vi "SwerveDriveCalibrate.vi"() -> ()   [LabVIEW 2014]
uses:
  <vilib>/Platform/TimedLoop/XDataNode/timing_clust.ctl
  <vilib>/Platform/TimedLoop/XDataNode/nitl_modes.ctl
  <vilib>/Platform/TimedLoop/XDataNode/wakeup.ctl
  <vilib>/Rock Robotics/WPI/CAN/TalonSRX/WPI_CANTalonSRX_APIControlMode.ctl
  <vilib>/Rock Robotics/WPI/CAN/TalonSRX/WPI_CANTalonSRX_APIFeedbackSelect.ctl
  <vilib>/Rock Robotics/WPI/SafetyOutput/WPI_SafetyOutputConfigMenu.ctl
  <vilib>/Rock Robotics/WPI/MotorControl/WPI_MotorControlOpenCANTalonSRX.vi
  <vilib>/Platform/TimedLoop/XDataNode/XDataNode.xnode
  <vilib>/Rock Robotics/WPI/MotorControl/WPI_MotorControlType.ctl
  <vilib>/Rock Robotics/SystemInterfaces/Typedef/FPGA_TypedefDigitalModule.ctl
  <vilib>/Rock Robotics/SystemInterfaces/DIO/FPGA_DIOPWMChannel.ctl
  <vilib>/Rock Robotics/WPI/PWM/WPI_PWMDeadband.ctl
  <vilib>/Rock Robotics/WPI/CAN/Jaguar/SubVIs/WPI_CANJaguar_ControlMode.ctl
  <vilib>/Rock Robotics/WPI/PWM/WPI_PWMTransform_ConPane.ctl
  <vilib>/Rock Robotics/WPI/MotorControl/WPI_MotorControlDeviceRef.ctl
  <vilib>/Platform/TimedLoop/XDataNode/XDNodeRunTimeDep.lvlib
panel:
  out "Analog In":dbl
  out "Encoder Position (-SRX)":dbl
  out "Sensor Position":dbl
  out "Quad velocities":dbl[](array[numeric])
  in  "Speed %VBus":dbl(slide) scale=-0.5..0.5
  out "Wheel Position":dbl(knob) scale=3.1416..-3.1416
  in  "Motor Controller":T1(ring)
  out "Waveform Chart":cluster{dbl, "motor output angle":dbl}(graph)
  in  "Enable":bool
  in  "Target Angle":dbl(knob) scale=3.1416..-3.1416
  in  "Offset":dbl
  in  "TPR":dbl=162.974661726
  in  "Set":bool
  in  "stop":bool
  out "error out":errorcluster
  in  "Steering PID":cluster{"P":dbl, "I":dbl, "D":dbl}
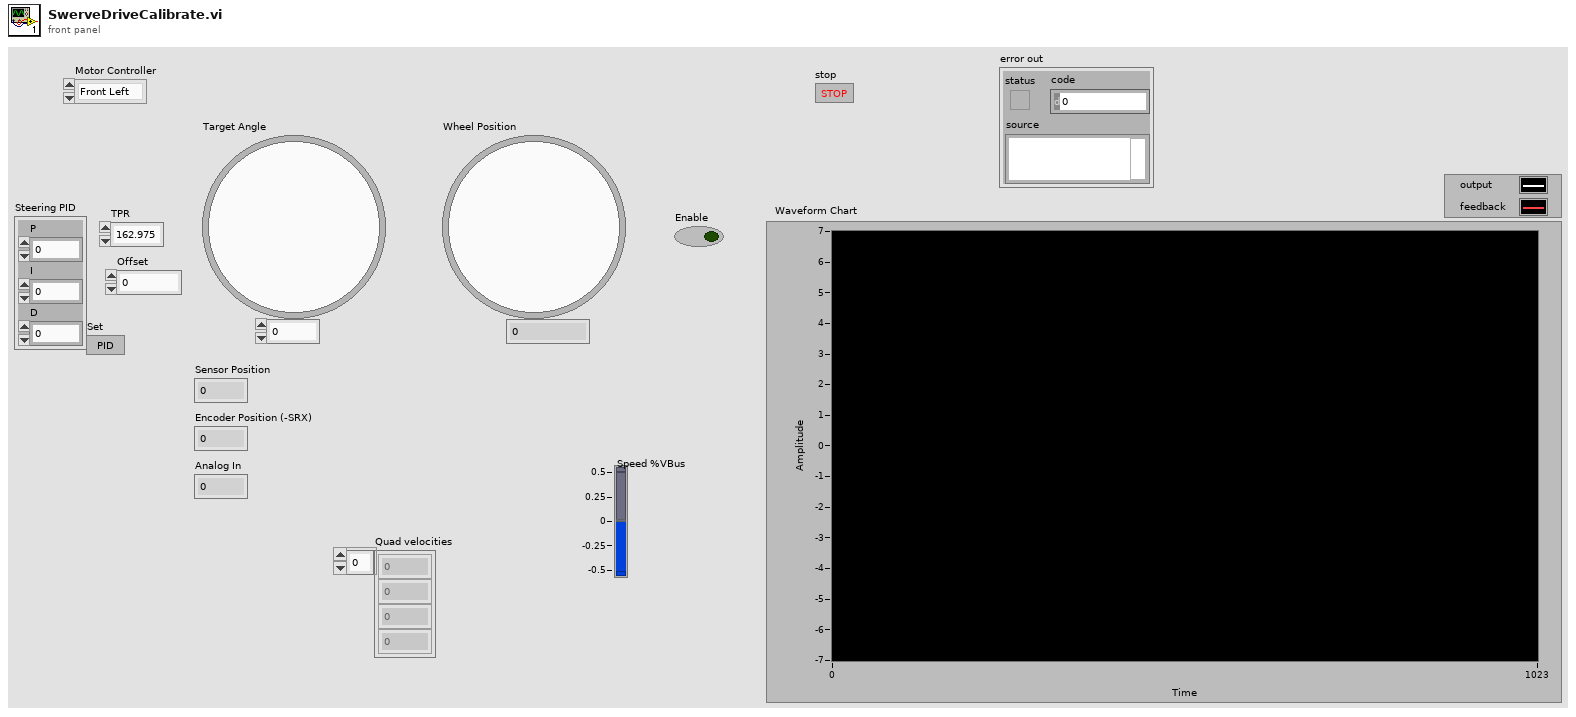
[diagram p1: front panel]
types:
  T1 = enum16{"Front Left", "Front Right", "Rear Left", "Rear Right"}
  T2 = typedef "WPI_MotorControlDeviceRef.ctl" = cluster{"DeviceStatus":errorcluster, "Type":T3, "PWM":cluster{"Controller":T4, "PWM Channel":T5, "DeadBand":T6}, "CAN":cluster{"Device Number":u8, "Control Mode":T7, "Semaphore":T8, "Max Vout":dbl, "TalonSRX Control Mode":T9}, "Invert":bool, "TransformRef":T10, "InvTransformRef":T10}
  T3 = typedef "WPI_MotorControlType.ctl" = enum16{"PWM", "CAN", "CANTalonSRX"}
  T4 = typedef "FPGA_TypedefDigitalModule.ctl" = enum16{"Controller 1"}
  T5 = typedef "FPGA_DIOPWMChannel.ctl" = enum8{"PWM 0", "PWM 1", "PWM 2", "PWM 3", "PWM 4", "PWM 5", "PWM 6", "PWM 7", "PWM 8", "PWM 9", "PWM MXP 0", "PWM MXP 1", "PWM MXP 2", "PWM MXP 3", "PWM MXP 4", "PWM MXP 5", "PWM MXP 6", "PWM MXP 7", "PWM MXP 8", "PWM MXP 9", "Invalid"}
  T6 = typedef "WPI_PWMDeadband.ctl" = cluster{"Name":string, "maxPositivePwm":i32, "minPositivePwm":i32, "centerPwm":i32, "maxNegativePwm":i32, "minNegativePwm":i32, "angularRange":u16}
  T7 = typedef "WPI_CANJaguar_ControlMode.ctl" = enum8{"Percent VBus", "Current", "Speed", "Position", "Voltage"}
  T8 = typedef "Semaphore RefNum" = refnum<k1>
  T9 = typedef "WPI_CANTalonSRX_APIControlMode.ctl" = enum8{"Percent VBus", "Speed", "Position", "Slave", "Unchanged / Invalid"}
  T10 = typedef "WPI_PWMTransform_ConPane.ctl" = refnum<vi>
  T11 = typedef "WPI_CANTalonSRX_APIFeedbackSelect.ctl" = enum16{"Digital Quadrature Encoder", "Analog Potentiometer", "Analog Encoder"}
  T12 = typedef "WPI_SafetyOutputConfigMenu.ctl" = enum16{"Enable", "Disable"}
  T13 = typedef "WPI_CANTalonSRX_GlobalStatus.ctl" = cluster{"Applied Throttle":dbl, "Module Enabled":bool, "CAN Error":errorcluster, "Closed Loop Error":dbl, "Forward Limit Switch Closed":bool, "Reverse Limit Switch Closed":bool, "Sensor Position":dbl, "Sensor Velocity":dbl, "Current":dbl, "Sticky Fault - Over Temp":bool, "Sticky Fault - Under Voltage":bool, "Sticky Fault - Forward Limit":bool, "Sticky Fault - Reverse Limit":bool, "Sticky Fault - Forward Soft Limit":bool, "Sticky Fault - Reverse Soft Limit":bool, "Brake is Enabled":bool, "Encoder Position":dbl, "Encoder Velocity":dbl, "Encoder Index Count":dbl, "Encoder A Pin State":bool, "Encoder B Pin State":bool, "Encoder Index Pin State":bool, "Analog In":dbl, "Analog In Velocity":dbl, "Temperature (C)":dbl, "Battery Voltage":dbl}
  T14 = typedef "XDNodeRunTimeDep.lvlib/timing_clust.ctl" = cluster{"Expected End [f-1]":u64, "Actual End [f-1]":u64, "Finished Late? [f-1]":bool, "Expected End [i-1]":u64, "Actual End [i-1]":u64, "Finished Late? [i-1]":bool, "Expected Start [i]":u64, "Actual Start [i]":u64, "Expected Start [f]":u64, "Actual Start [f]":u64, "Source Name":string, "Structure Name":string, "Period":i64, "Deadline":i64, "Offset":i64, "Start":i64, "Priority":i32, "Timeout":i32, "Mode":T15, "Wakeup Reason":T16, "Error":errorcluster, "Source Type":string, "Secondary Source Type":string, "Global End Time":u64, "Global Start Time":u64, "Frame Duration":u64, "Iteration Duration":u64, "Assigned CPU":i32, "I/O Scan Engine Mode":u32}
  T15 = typedef "XDNodeRunTimeDep.lvlib/nitl_modes.ctl" = enum32{"No Change", "Process missed periods, maintain original phase", "Discard missed periods, maintain original phase", "Process missed periods, ignore original phase", "Discard missed periods, ignore original phase"}
  T16 = typedef "XDNodeRunTimeDep.lvlib/wakeup.ctl" = enum32{"Normal", "Aborted", "Asynchronous wakeup", "Timing source error", "Timed loop error", "Timeout"}
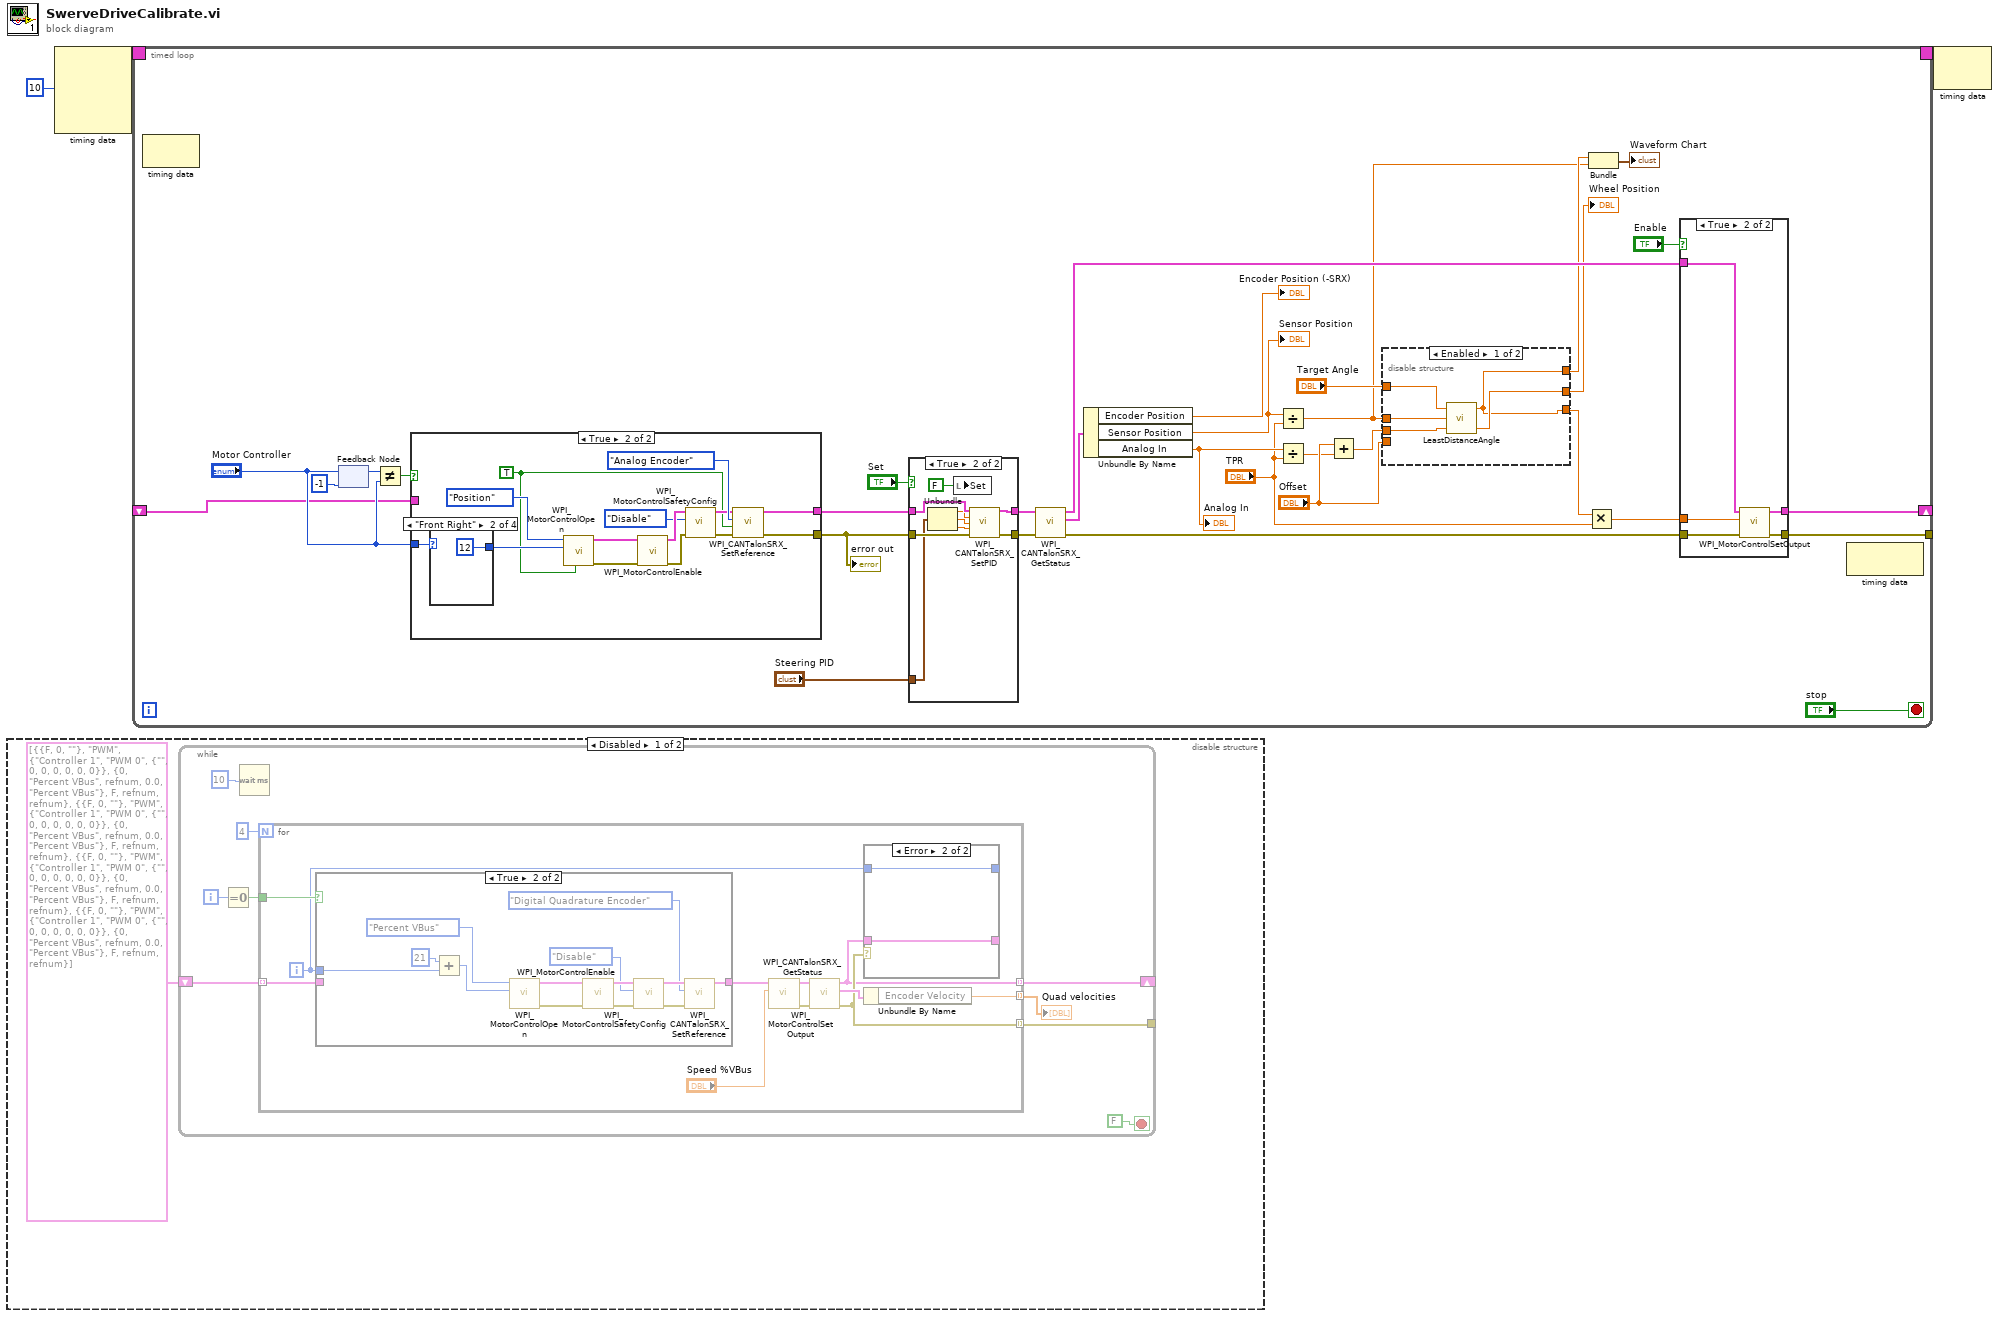
[diagram p0: block diagram]
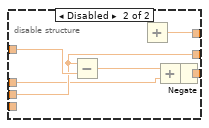
[diagram p5: hidden frame]
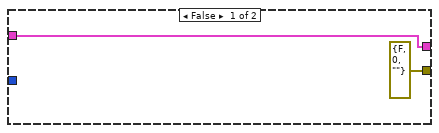
[diagram p6: hidden frame]
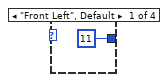
[diagram p7: hidden frame]
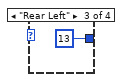
[diagram p8: hidden frame]
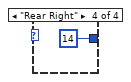
[diagram p9: hidden frame]
diagram:
  n1 = disable-structure shown="Disabled" {
    frame Disabled {
      n2 = while {
        shift-right: [w9] -> _
        shift-left: T2[] [{"DeviceStatus"={"status"=FALSE, "code"=0, "source"=""}, "Type"=enum."PWM", "PWM"={"Controller"=enum."Controller 1", "PWM Channel"=enum."PWM 0", "DeadBand"={"Name"="", "maxPositivePwm"=0, "minPositivePwm"=0, "centerPwm"=0, "maxNegativePwm"=0, "minNegativePwm"=0, "angularRange"=0}}, "CAN"={"Device Number"=0, "Control Mode"=enum."Percent VBus", "Semaphore"=refnum, "Max Vout"=0.0, "TalonSRX Control Mode"=enum."Percent VBus"}, "Invert"=FALSE, "TransformRef"=refnum, "InvTransformRef"=refnum}, {"DeviceStatus"={"status"=FALSE, "code"=0, "source"=""}, "Type"=enum."PWM", "PWM"={"Controller"=enum."Controller 1", "PWM Channel"=enum."PWM 0", "DeadBand"={"Name"="", "maxPositivePwm"=0, "minPositivePwm"=0, "centerPwm"=0, "maxNegativePwm"=0, "minNegativePwm"=0, "angularRange"=0}}, "CAN"={"Device Number"=0, "Control Mode"=enum."Percent VBus", "Semaphore"=refnum, "Max Vout"=0.0, "TalonSRX Control Mode"=enum."Percent VBus"}, "Invert"=FALSE, "TransformRef"=refnum, "InvTransformRef"=refnum}, {"DeviceStatus"={"status"=FALSE, "code"=0, "source"=""}, "Type"=enum."PWM", "PWM"={"Controller"=enum."Controller 1", "PWM Channel"=enum."PWM 0", "DeadBand"={"Name"="", "maxPositivePwm"=0, "minPositivePwm"=0, "centerPwm"=0, "maxNegativePwm"=0, "minNegativePwm"=0, "angularRange"=0}}, "CAN"={"Device Number"=0, "Control Mode"=enum."Percent VBus", "Semaphore"=refnum, "Max Vout"=0.0, "TalonSRX Control Mode"=enum."Percent VBus"}, "Invert"=FALSE, "TransformRef"=refnum, "InvTransformRef"=refnum}, {"DeviceStatus"={"status"=FALSE, "code"=0, "source"=""}, "Type"=enum."PWM", "PWM"={"Controller"=enum."Controller 1", "PWM Channel"=enum."PWM 0", "DeadBand"={"Name"="", "maxPositivePwm"=0, "minPositivePwm"=0, "centerPwm"=0, "maxNegativePwm"=0, "minNegativePwm"=0, "angularRange"=0}}, "CAN"={"Device Number"=0, "Control Mode"=enum."Percent VBus", "Semaphore"=refnum, "Max Vout"=0.0, "TalonSRX Control Mode"=enum."Percent VBus"}, "Invert"=FALSE, "TransformRef"=refnum, "InvTransformRef"=refnum}] -> [w8]
        tunnel: [w6] -> _
        i -> [w12]
        stop <- FALSE stop-if-true
        n3 = Equal To 0?(x=w12) -> (x = 0?=w10:bool)
        n4 = Wait (ms)(milliseconds to wait=u32 10) -> ()  [unwired: 1 out]
        n5 = for {
          N: 4 -> [_]
          tunnel: w10 -> [w24]
          tunnel: [w14] -> w9 mode=indexing
          tunnel: w8 -> [w23] mode=indexing
          tunnel: [w16] -> w6 mode=indexing
          tunnel: [w17] -> w5 mode=indexing
          i -> [w15]
          n6 = case shown="True" w24 {
            tunnel: [w29 w31] -> w22
            tunnel: w23 -> [w29 _]
            tunnel: w15 -> [_ w35]
            frame False {
            }
            frame True {
              n7 = Add(x=21, y=w35) -> (x+y=w34:i32)
              n8 = call-poly <vilib>:"WPI_MotorControlOpen.vi"("Device Number"=w34, "Control Mode"=WPI_CANTalonSRX_APIControlMode."Percent VBus") -> ("error out"=w41:errorcluster, "MotorControlDeviceRef"=w40:T2)  [unwired: 8 in]
              n9 = call <vilib>:"WPI_MotorControlEnable.vi"("error in (no error)"=w41, "CAN Jaguar Ref"=w40) -> ("error out"=w38:errorcluster, "CAN Jaguar Ref Out"=w39:T2)  [unwired: 8 in]
              n10 = call <vilib>:"WPI_MotorControlSafetyConfig.vi"("error in (no error)"=w38, "mode"=WPI_SafetyOutputConfigMenu."Disable", "MotorControlDevRef"=w39) -> ("error out"=w32:errorcluster, "MotorControlDevRef"=w33:T2)  [unwired: 7 in]
              n11 = call <vilib>:"WPI_CANTalonSRX_SetReference.vi"("error in (no error)"=w32, "Feedback Reference"=WPI_CANTalonSRX_APIFeedbackSelect."Digital Quadrature Encoder", "CAN Talon SRX Ref"=w33) -> ("CAN Talon SRX Ref Out"=w31:T2)  [unwired: 7 in, 1 out]
            }
          }
          n12 = call <vilib>:"WPI_MotorControlSetOutput.vi"("Output"="Speed %VBus", "MotorControlDevRef"=w22) -> ("error out"=w20:errorcluster, "MotorControlDevRef"=w19:T2)  [unwired: 7 in, 1 out]
          n13 = call <vilib>:"WPI_CANTalonSRX_GetStatus.vi"("error in (no error)"=w20, "CAN Talon SRX Ref"=w19) -> ("error out"=w16:errorcluster, "Talon SRX Status"=w18:T13, "CAN Talon SRX Ref Out"=w14:T2)  [unwired: 7 in]
          n14 = case shown="Error" w16 {
            tunnel: [w26 w27] -> _
            tunnel: w15 -> [w26 w27]
            tunnel: [w25 w28] -> _
            tunnel: w14 -> [w25 w28]
            frame No Error {
            }
            frame Error {
            }
          }
          n15 = Unbundle By Name(w18) -> ("Encoder Velocity"=w17:dbl)
        }
        "Quad velocities" <- w5
      }
    }
    frame Enabled {
    }
  }
  n16 = node-c288(i64 10 ("Period")) -> (w3:T14)  [unwired: 3 in]
  n17 = timed-loop {
    timing: w3 -> [_]
    timing-out: [_] -> w2
    shift-right: [w62] -> _
    shift-left: _ -> [w54]
    tunnel: [w49] -> _
    stop <- "stop" stop-if-true
    n18 = node-c288() -> ()  [unwired: 1 in, 1 out]
    n19 = feedback-in #1("Motor Controller") -> ()
    n20 = feedback #1(-1) -> (w59:i32)
    n21 = Not Equal?(x=w59, y="Motor Controller") -> (x != y?=w56:bool)
    n22 = case shown="True" w56 {
      tunnel: "Motor Controller" -> [_ w97]
      tunnel: [w88 w96] -> w61
      tunnel: [errorcluster {"status"=FALSE, "code"=0, "source"=""} ("error out") w95] -> w60
      tunnel: w54 -> [w88 _]
      frame False {
      }
      frame True {
        w89 = TRUE ("Invert")
        n23 = case shown="\"Front Right\"" w97 {
          tunnel: [11 12 13 14] -> w99
          frame "Front Left", Default {
          }
          frame "Front Right" {
          }
          frame "Rear Left" {
          }
          frame "Rear Right" {
          }
        }
        n24 = call-poly <vilib>:"WPI_MotorControlOpen.vi"("Invert"=w89, "Device Number"=w99, "Control Mode"=WPI_CANTalonSRX_APIControlMode."Position") -> ("error out"=w101:errorcluster, "MotorControlDeviceRef"=w100:T2)  [unwired: 7 in]
        n25 = call <vilib>:"WPI_MotorControlEnable.vi"("error in (no error)"=w101, "CAN Jaguar Ref"=w100) -> ("error out"=w93:errorcluster, "CAN Jaguar Ref Out"=w94:T2)  [unwired: 8 in]
        n26 = call <vilib>:"WPI_MotorControlSafetyConfig.vi"("error in (no error)"=w93, "mode"=WPI_SafetyOutputConfigMenu."Disable", "MotorControlDevRef"=w94) -> ("error out"=w92:errorcluster, "MotorControlDevRef"=w91:T2)  [unwired: 7 in]
        n27 = call <vilib>:"WPI_CANTalonSRX_SetReference.vi"("error in (no error)"=w92, "Reverse Feedback Sensor"=w89, "Feedback Reference"=WPI_CANTalonSRX_APIFeedbackSelect."Analog Encoder", "CAN Talon SRX Ref"=w91) -> ("error out"=w95:errorcluster, "CAN Talon SRX Ref Out"=w96:T2)  [unwired: 6 in]
      }
    }
    "error out" <- w60
    n28 = case shown="True" "Set" {
      tunnel: w61 -> [w115 w123]
      tunnel: w60 -> [w114 w122]
      tunnel: [w114 w121] -> w71
      tunnel: [w115 w120] -> w70
      tunnel: "Steering PID" -> [_ w116]
      frame False {
      }
      frame True {
        n29 = Unbundle(w116) -> ("P"=w119:dbl, "I"=w118:dbl, "D"=w117:dbl)
        n30 = local write "Set"(FALSE) -> ()
        n31 = call <vilib>:"WPI_CANTalonSRX_SetPID.vi"("CAN Talon SRX Ref"=w123, "P"=w119, "I"=w118, "D"=w117, "error in (no error)"=w122) -> ("CAN Talon SRX Ref Out"=w120:T2, "error out"=w121:errorcluster)  [unwired: 9 in]
      }
    }
    n32 = call <vilib>:"WPI_CANTalonSRX_GetStatus.vi"("error in (no error)"=w71, "CAN Talon SRX Ref"=w70) -> ("error out"=w67:errorcluster, "Talon SRX Status"=w73:T13, "CAN Talon SRX Ref Out"=w66:T2)  [unwired: 7 in]
    n33 = Unbundle By Name(w73) -> ("Encoder Position"=→"Encoder Position (-SRX)":dbl, "Sensor Position"=w46:dbl, "Analog In"=w72:dbl)
    "Sensor Position" <- w46
    "Analog In" <- w72
    n34 = Divide(x=w46, y="TPR") -> (x/y=w43:dbl)
    n35 = Divide(x=w72, y="TPR") -> (x/y=w53:dbl)
    n36 = Add(x="Offset", y=w53) -> (x+y=w51:dbl)
    n37 = disable-structure shown="Enabled" {
      disable-tunnel: "Offset" -> [_ _]
      disable-tunnel: [w75 w81] -> w68
      disable-tunnel: "Target Angle" -> [w79 w86]
      disable-tunnel: w51 -> [w78 w84]
      disable-tunnel: [w77 w84] -> w50
      disable-tunnel: [w75 w80] -> w48
      disable-tunnel: w43 -> [w76 w82]
      frame Enabled {
        n38 = call "LeastDistanceAngle.vi"("current angle (no limits)"=w78, "Sensor position"=w76, "target angle (between pi and -pi)"=w79) -> ("current angle (between pi and -pi)"=w77:dbl, "motor output angle"=w75:dbl)  [unwired: 1 out]
      }
      frame Disabled {
        n39 = Subtract(x=w84, y=w86) -> (x-y=w83:dbl)
        n40 = Add() -> (x+y=w80:dbl)  [unwired: 2 in]
        n41 = Add(x=w83, y=w82) -> (x+y=w85:dbl)
        n42 = Negate(x=w85) -> (-x=w81:dbl)
      }
    }
    "Wheel Position" <- w50
    n43 = Multiply(x=w68, y="TPR") -> (x*y=w44:dbl)
    n44 = Bundle("motor output angle"=w48, w43) -> (→"Waveform Chart":cluster{"motor output angle":dbl, dbl})  [unwired: 1 in]
    n45 = case shown="True" "Enable" {
      tunnel: w67 -> [w108 w113]
      tunnel: [w108 w112] -> w49
      tunnel: w66 -> [w107 w111]
      tunnel: [w107 w110] -> w62
      tunnel: w44 -> [_ w109]
      frame False {
      }
      frame True {
        n46 = call <vilib>:"WPI_MotorControlSetOutput.vi"("error in (no error)"=w113, "Output"=w109, "MotorControlDevRef"=w111) -> ("error out"=w112:errorcluster, "MotorControlDevRef"=w110:T2)  [unwired: 6 in, 1 out]
      }
    }
    n47 = node-c288() -> ()  [unwired: 1 in, 1 out]
  }
  n48 = node-c288(w2) -> ()  [unwired: 1 out]
